vi "Cleanup.vi"(8 "error in (no error)":errorcluster, 11 "Prototyper in":refnum<class "Prototyper.lvclass">) -> (0 "error out":errorcluster, 3 "Prototyper out":refnum<class "Prototyper.lvclass">)   [LabVIEW 2020, in "Message Maker.lvlib" / "Prototyper.lvclass"]
uses:
  Prototyper.lvclass
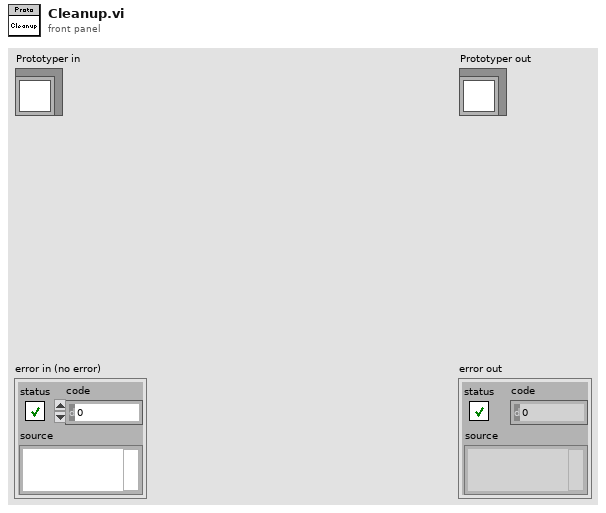
[diagram p1: front panel]
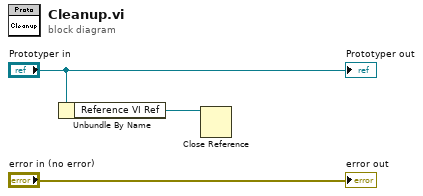
[diagram p0: block diagram]
diagram:
  n1 = Unbundle By Name("Prototyper in") -> ("Reference VI Ref"=w2:refnum<vi>)
  n2 = Close Reference(reference=w2) -> ()  [unwired: 1 in, 1 out]
  "error out" <- "error in (no error)"
  "Prototyper out" <- "Prototyper in"
